vi "Unsigned to Binary.vi"(1 "UInt In":i32[](array[numeric]), 2 "QAM Complexity":T1(ring)) -> (0 "BitStream Out":i32[](array[numeric]))   [LabVIEW 2018]
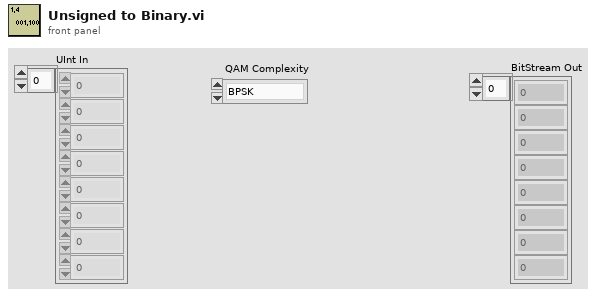
[diagram p1: front panel]
types:
  T1 = enum16{"BPSK", "QPSK", "16-QAM", "64-QAM", "256-QAM"}
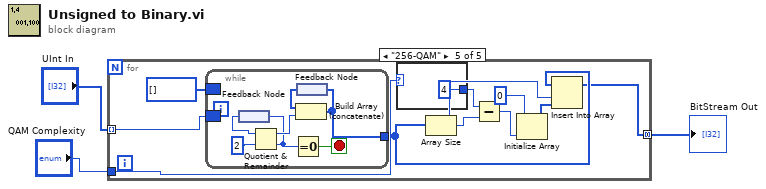
[diagram p0: block diagram]
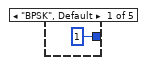
[diagram p2: hidden frame]
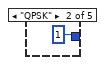
[diagram p3: hidden frame]
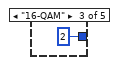
[diagram p4: hidden frame]
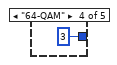
[diagram p5: hidden frame]
diagram:
  n1 = for {
    tunnel: "UInt In" -> [w5] mode=indexing
    tunnel: [w6] -> w2 mode=concatenating
    tunnel: "QAM Complexity" -> [w11]
    n2 = while {
      border: i32[] [] -> [_]
      tunnel: [w22] -> w7
      border: w5 -> [_]
      stop <- w24 stop-if-true
      n3 = feedback #1() -> (w20:i32)
      n4 = Quotient & Remainder(x=w20, y=2) -> (x-y*floor(x/y)=w21:i32, floor(x/y)=w19:i32)
      n5 = feedback-in #1(w19) -> ()
      n6 = Equal To 0?(x=w19) -> (x = 0?=w24:bool)
      n7 = feedback #2() -> (w23:i32[])
      n8 = Build Array (concatenate)(w23, w21) -> (w22:i32[])
      n9 = feedback-in #2(w22) -> ()
    }
    n10 = case shown="\"256-QAM\"" w11 {
      tunnel: [1 1 2 3 4] -> w12
      frame "BPSK", Default {
      }
      frame "QPSK" {
      }
      frame "16-QAM" {
      }
      frame "64-QAM" {
      }
      frame "256-QAM" {
      }
    }
    n11 = Array Size(array=w7) -> (size(s)=w4:i32)
    n12 = Subtract(x=w12, y=w4) -> (x-y=w10:i32)
    n13 = Initialize Array(0 ("element"), w10) -> (w8:i32[])
    n14 = Insert Into Array(array=w7, index=w4, new element=w8) -> (w6:i32[])
  }
  "BitStream Out" <- w2
